vi "whileLoopSample.vi"() -> ()   [LabVIEW 2025]
doc: "Uses a While Loop to compare two numbers for equality. For each comparison, a boolean value (True or False) is generated and stored in a boolean array, indicating whether the numbers are equal at each iteration."
panel:
  out "boolean array":bool[](array[boolean])
  in  "a1":dbl
  in  "b1":dbl
  in  "?":bool
  out "equality check":bool
  # "Sample while loop for equality of 2 numbers and generating boolean array for each check"
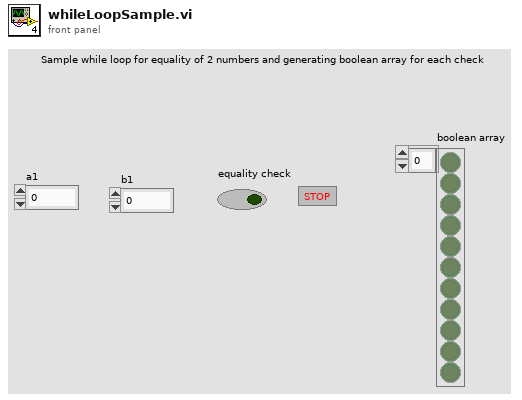
[diagram p1: front panel]
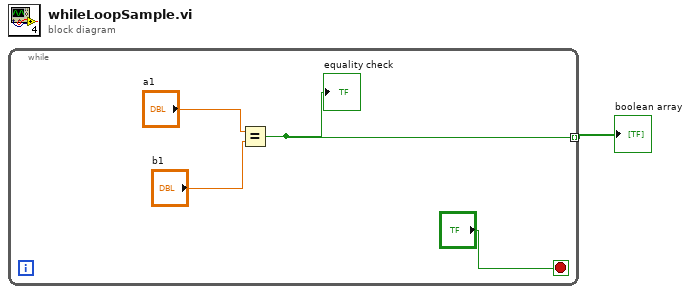
[diagram p0: block diagram]
diagram:
  n1 = while {
    tunnel: [w2] -> w1 mode=indexing
    stop <- "?" stop-if-true
    n2 = Equal?(x="a1", y="b1") -> (x = y?=w2:bool)
    "equality check" <- w2
  }
  "boolean array" <- w1
